vi "Convert Frame Array to String Array.vi"(11 "Array in":T1[](array[typedef]) {"payload" format="%x"; "timestamp" format="%<%.7X\n%x>T"; "type" items=["CAN Data"=0, "CAN Remote"=1, "CAN Bus Error"=2, "CAN 2.0 Data"=8, "CAN FD Data"=16, "CAN FD+BRS Data"=24, "J1939 Data"=192, "Delay"=224, "Log Trigger"=225, "Start Trigger"=226]; "identifier" format="%x"}) -> (3 "Array out":string[][](array[string]))   [LabVIEW 2019, in "CAN Stream Support Workspace Shared.lvlib"]
uses:
  CAN Stream Support Workspace Shared.lvlib
  <vilib>/xnet/xnet.llb/XNET Frame CAN.ctl
  <vilib>/xnet/xnet.llb/XNET Frame Type CAN.ctl
  <vilib>/Utility/error.llb/Trim Whitespace One-Sided.vi
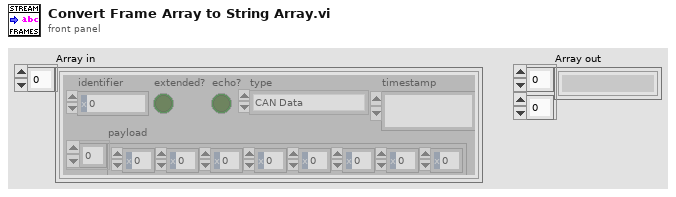
[diagram p1: front panel]
types:
  T1 = typedef "XNET Frame CAN.ctl" = cluster{"timestamp":timestamp, "payload":u8[], "identifier":u32, "type":T2, "extended?":bool, "echo?":bool}
  T2 = typedef "XNET Frame Type CAN.ctl" = u8
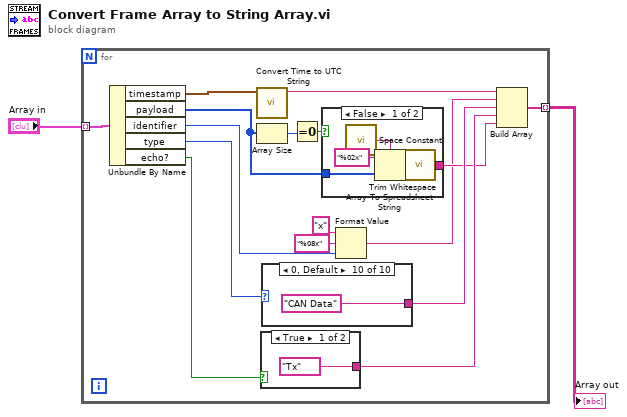
[diagram p0: block diagram]
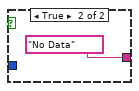
[diagram p2: hidden frame]
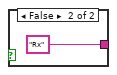
[diagram p3: hidden frame]
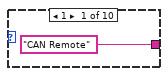
[diagram p4: hidden frame]
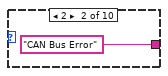
[diagram p5: hidden frame]
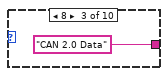
[diagram p6: hidden frame]
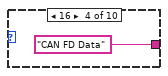
[diagram p7: hidden frame]
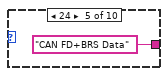
[diagram p8: hidden frame]
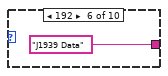
[diagram p9: hidden frame]
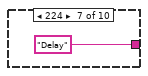
[diagram p10: hidden frame]
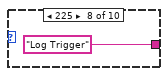
[diagram p11: hidden frame]
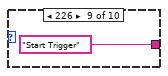
[diagram p12: hidden frame]
diagram:
  n1 = for {
    tunnel: "Array in" -> [w18] mode=indexing
    tunnel: [w6] -> w1 mode=indexing
    n2 = Unbundle By Name(w18) -> ("timestamp"=w17:timestamp, "payload"=w10:u8[], "identifier"=w16:u32, "type"=w15:T2, "echo?"=w13:bool)
    n3 = call "Convert Time to UTC String.vi"("timestamp"=w17) -> ("UTC string"=w8:string)  [unwired: 10 in]
    n4 = Array Size(array=w10) -> (size(s)=w12:i32)
    n5 = case shown="True" w13 {
      tunnel: ["Tx" "Rx"] -> w9
      frame True {
      }
      frame False {
      }
    }
    n6 = case shown="0, Default" w15 {
      tunnel: ["CAN Remote" "CAN Bus Error" "CAN 2.0 Data" "CAN FD Data" "CAN FD+BRS Data" "J1939 Data" "Delay" "Log Trigger" "Start Trigger" "CAN Data"] -> w14
      frame 1 {
      }
      frame 2 {
      }
      frame 8 {
      }
      frame 16 {
      }
      frame 24 {
      }
      frame 192 {
      }
      frame 224 {
      }
      frame 225 {
      }
      frame 226 {
      }
      frame 0, Default {
      }
    }
    n7 = Equal To 0?(x=w12) -> (x = 0?=w11:bool)
    n8 = case shown="False" w11 {
      tunnel: [w19 "No Data"] -> w7
      tunnel: w10 -> [w23 _]
      frame False {
        n9 = call <vilib>:"Space Constant.vi"() -> ("String"=w20:string)
        n10 = Array To Spreadsheet String(delimiter (Tab)=w20, array=w23, 3:"%02x" ("format string")) -> (spreadsheet string=w22:string)
        n11 = call <vilib>:"Trim Whitespace.vi"("string"=w22) -> ("trimmed string"=w19:string)  [unwired: 1 in]
      }
      frame True {
      }
    }
    n12 = Format Value(string ("")="x" ("string"), format string="%08x", value (0)=w16) -> (output string=w3:string)
    n13 = Build Array(w8, w3, w14, w9, w7) -> (w6:string[])
  }
  "Array out" <- w1
